vi "LIA_DAQ_SetModuleParameters.vi"(8 "error in (no error)":errorcluster, 10 "LIA DAQ Module Parameters":T2[](array[typedef]) {"Value" format="%#_6p"}, 11 "DAQ ModHandle In":T1 {"ModHandle" format="0x%08x"; "Conn" format="0x%08x"}) -> (0 "error out":errorcluster, 3 "DAQ ModHandle Out":T1 {"ModHandle" format="0x%08x"; "Conn" format="0x%08x"})   [LabVIEW 2016, in "ZI LIA.lvlib"]
uses:
  ZI LIA.lvlib
  Ctl_SetParameter(Value).ctl
  <instrlib>/Zurich Instruments LabOne/Public/Modules/ziTypeModHandle.ctl
  <instrlib>/Zurich Instruments LabOne/Public/Modules/ziModSetValueDoubleArray.vi
  <instrlib>/Zurich Instruments LabOne/Zurich Instruments LabOne.lvlib
  General.lvlib
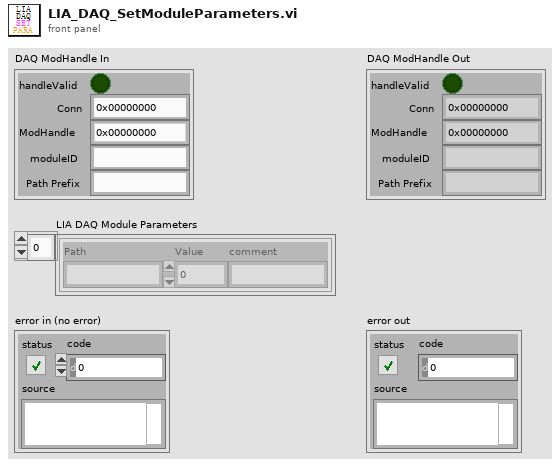
[diagram p1: front panel]
types:
  T1 = typedef "Zurich Instruments LabOne.lvlib/ziTypeModHandle.ctl" = cluster{"handleValid":bool, "Conn":u64, "ModHandle":u64, "moduleID":string, "Path Prefix":string}
  T2 = typedef "General.lvlib/Ctl_SetParameter(Value).ctl" = cluster{"Path":string, "Value":dbl, "comment":string}
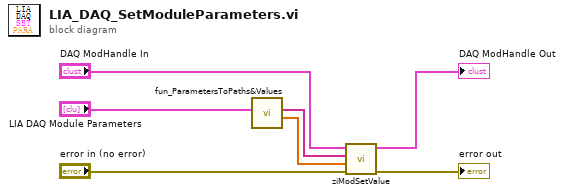
[diagram p0: block diagram]
diagram:
  n1 = call "fun_ParametersToPaths&Values.vi"("Parameters"="LIA DAQ Module Parameters") -> ("Values"=w7:dbl[], "Paths"=w6:string[])  [unwired: 9 in]
  n2 = call-poly <instrlib>:"ziModSetValue.vi"("Error In"="error in (no error)", "Values"=w7, "Paths"=w6, "ModHandle In"="DAQ ModHandle In") -> ("Error Out"=→"error out":errorcluster, "ModHandle Out"=→"DAQ ModHandle Out":T1)  [unwired: 6 in]
